vi "layout.vi"(0 "reference":refnum<class "ChoiceNode.lvclass">, 1 "graph":refnum<class "Graph.lvclass">, 2 "graphics":refnum<class "Graphics.lvclass">, 3 "grid":refnum<class "Grid.lvclass">, 5 "error in (no error)":errorcluster) -> (14 "reference out":refnum<class "ChoiceNode.lvclass">, 19 "error out":errorcluster)   [LabVIEW 2012, in "ChoiceNode.lvclass"]
doc: "public void layout(Graph g, Graphics2D g2, Grid grid)"
uses:
  <resource>/Framework/Providers/Open_GDS/UML/ChoiceNode_class/ChoiceNode.lvclass
  <resource>/Framework/Providers/Open_GDS/UML/Graph_class/Graph.lvclass
  <resource>/Framework/Providers/Open_GDS/UML/Graphics_class/Graphics.lvclass
  <resource>/Framework/Providers/Open_GDS/UML/Grid_class/Grid.lvclass
  <resource>/Framework/Providers/Open_GDS/UML/General/Rectangle/Rectangle Rectangle2D.ctl
  <resource>/Framework/Providers/Open_GDS/UML/MultiLineString_class/MultiLineString.lvclass
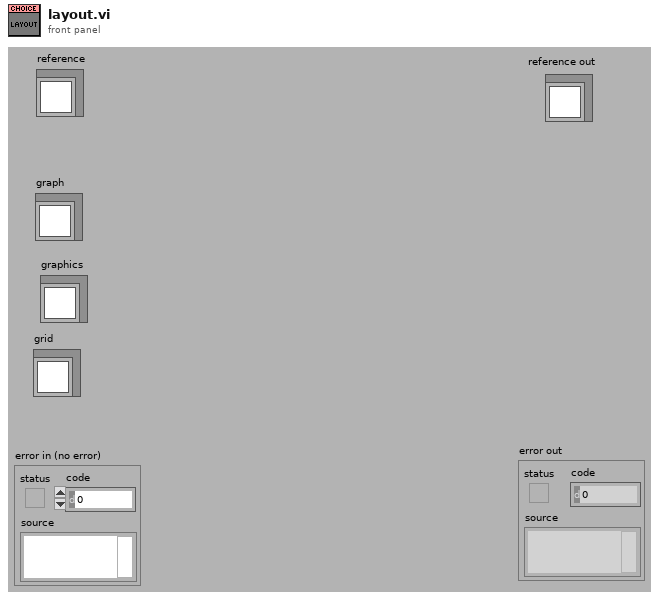
[diagram p1: front panel]
types:
  T1 = typedef "Rectangle Rectangle2D.ctl" = cluster{"x":dbl, "y":dbl, "width":dbl, "height":dbl}
  T2 = typedef "ChoiceNode.lvclass/ObjectAttributes.ctl" = cluster{"Base class":T3, "Text":refnum<class "MultiLineString.lvclass">, "DEFAULT_WIDTH":i32, "DEFAULT_HEIGHT":i32}
  T3 = typedef "RectangularNode.lvclass/ObjectAttributes.ctl" = cluster{"Base class":T4, "bounds":T1}
  T4 = typedef "AbstractNode.lvclass/ObjectAttributes.ctl" = cluster{"parent":refnum<class "AbstractNode.lvclass">, "children":refnum<class "AbstractNode.lvclass">[], "Hidden":bool}
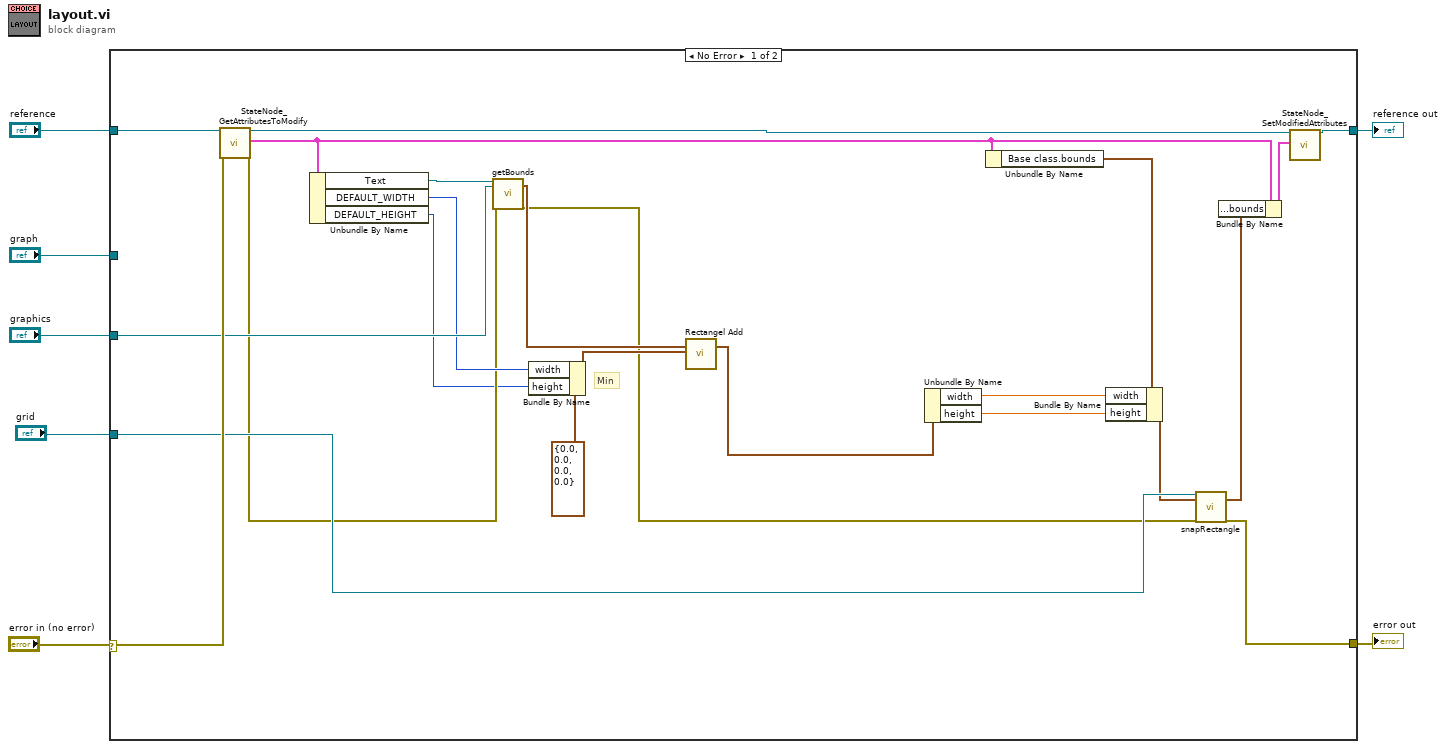
[diagram p0: block diagram]
diagram:
  n1 = case shown="No Error" "error in (no error)" {
    selector: "error in (no error)" -> [w27 w31]
    tunnel: "reference" -> [w30 w32]
    tunnel: [w29 w31] -> w6
    tunnel: [w28 w32] -> w5
    tunnel: "graph" -> [_ _]
    tunnel: "graphics" -> [w26 _]
    tunnel: "grid" -> [w25 _]
    frame No Error {
      # "Min"
      n2 = call <resource>:"StateNode_GetAttributesToModify.vi"("reference in"=w30, "error in (no error)"=w27) -> ("reference out"=w15:refnum<class "ChoiceNode.lvclass">, "Attributes"=w19:T2, "error out"=w16:errorcluster)  [unwired: 1 in, 14 out]
      n3 = Unbundle By Name(w19) -> ("Text"=w24:refnum<class "MultiLineString.lvclass">, "DEFAULT_WIDTH"=w23:i32, "DEFAULT_HEIGHT"=w12:i32)
      n4 = call-dynamic "getBounds.vi"("reference"=w24, "graphics"=w26, "error in (no error)"=w16) -> ("bounds"=w10:T1, "error out"=w9:errorcluster)  [unwired: 15 out]
      n5 = Bundle By Name(cluster=T1 {"x"=0.0, "y"=0.0, "width"=0.0, "height"=0.0} ("bounds"), "width"=w23, "height"=w12) -> (w13:T1)
      n6 = call <resource>:"Rectangel Add.vi"("bounds1"=w10, "bounds2"=w13) -> ("boundsAdded"=w11:T1)  [unwired: 3 in, 14 out]
      n7 = Unbundle By Name(w11) -> ("width"=w21:dbl, "height"=w8:dbl)
      n8 = Unbundle By Name(w19) -> ("Base class.bounds"=w20:T1)
      n9 = Bundle By Name(cluster=w20, "width"=w21, "height"=w8) -> (w18:T1)
      n10 = call <resource>:"snapRectangle.vi"("reference"=w25, "bounds"=w18, "error in (no error)"=w9) -> ("boundsOut"=w17:T1, "error out"=w29:errorcluster)  [unwired: 15 out]
      n11 = Bundle By Name(cluster=w19, "Base class.bounds"=w17) -> (w14:T2)
      n12 = call <resource>:"StateNode_SetModifiedAttributes.vi"("reference in"=w15, "Attributes"=w14) -> ("reference out"=w28:refnum<class "ChoiceNode.lvclass">)  [unwired: 4 in, 13 out]
    }
    frame Error {
    }
  }
  "reference out" <- w5
  "error out" <- w6
